vi "Get DIO Bits For Jog Mode Assignement.vi"(4 "error in (no error)":errorcluster, 6 "Axis (1)":i32=1 min=1 max=3, 7 "VISA resource name":refnum<visa-resource-name>) -> (0 "error out":errorcluster, 1 "Bit# for positive direction":i32, 2 "Bit# for negative direction":i32, 3 "VISA resource name out":refnum<visa-resource-name>)   [LabVIEW 2020, in "Newport ESP301.lvlib"]
doc: "Get the DIO bits used for jogging in negative and positive directions respectively"
uses:
  Newport ESP301.lvlib
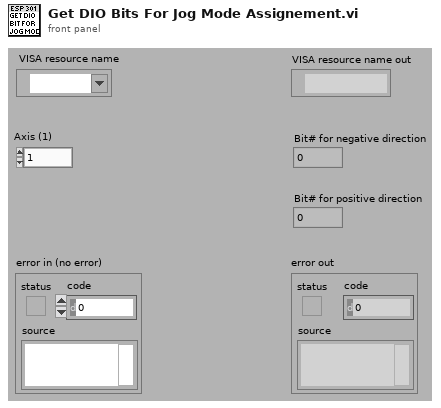
[diagram p1: front panel]
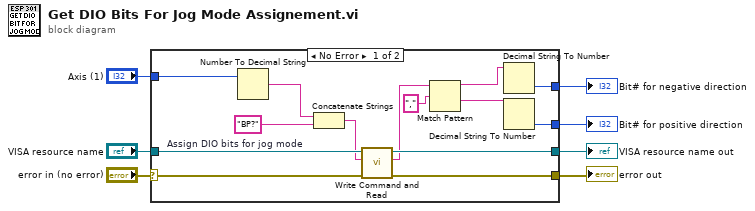
[diagram p0: block diagram]
diagram:
  n1 = case shown="No Error" "error in (no error)" {
    selector: "error in (no error)" -> [w20 w23]
    tunnel: [w12 w23] -> w7
    tunnel: "VISA resource name" -> [w21 w22]
    tunnel: [w15 w22] -> w6
    tunnel: "Axis (1)" -> [w17 _]
    tunnel: [w14 _] -> w2
    tunnel: [w13 _] -> w1
    frame No Error {
      w18 = "BP?"  # Assign DIO bits for jog mode
      n2 = Number To Decimal String(number=w17) -> (decimal integer string=w19:string)  [unwired: 1 out]
      n3 = Concatenate Strings(w19, w18) -> (w16:string)
      n4 = call "Write Command and Read.vi"("error in (no error)"=w20, "Command"=w16, "VISA resource name"=w21) -> ("error out"=w12:errorcluster, "Returned string"=w10:string, "VISA resource name out"=w15:refnum<visa-resource-name>)  [unwired: 2 in, 2 out]
      n5 = Match Pattern(string=w10, regular expression="," ("search string/char (-)")) -> (before substring=w8:string, after substring=w9:string)  [unwired: 1 in, 2 out]
      n6 = Decimal String To Number(string=w8) -> (number=w14:i32)  [unwired: 1 in, 2 out]
      n7 = Decimal String To Number(string=w9) -> (number=w13:i32)  [unwired: 1 in, 2 out]
    }
    frame Error {
    }
  }
  "error out" <- w7
  "VISA resource name out" <- w6
  "Bit# for negative direction" <- w2
  "Bit# for positive direction" <- w1
